vi "SCCAPI Initialize.vi"(8 "error in (no error)":errorcluster, 10 "provider location":string, 11 "providerName":string) -> (0 "error out":errorcluster, 2 "suppCaps":u32)   [LabVIEW 2017, in "NI_SCC.lvlib"]
uses:
  <vilib>/SourceControl/sccapi/NI_SCC.lvlib
  <vilib>/SourceControl/sccapi/SCCAPI SCC Operations.ctl
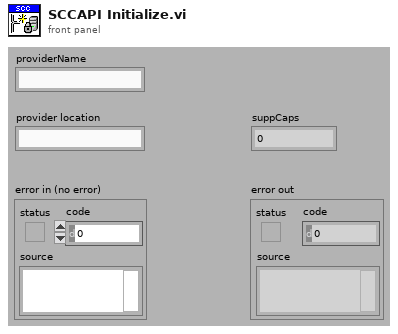
[diagram p1: front panel]
types:
  T1 = typedef "NI_SCC.lvlib/SCCAPI SCC Operations.ctl" = enum16{"Add", "Check In", "Check Out", "Close Project", "Compare Files", "Compare VIs", "Configure Project", "File History", "File Properties", "File Status", "Find All Providers", "Get Advanced Command Options", "Get File Copy", "Get Latest Version", "Get Project Name", "Get StaticVI Path", "Initialize", "Not A Source Control Reference", "Open Project", "Provider Supports Functionality", "Remove", "Run Provider", "Undo Check Out", "Uninitialize", "Is File In Local Path"}
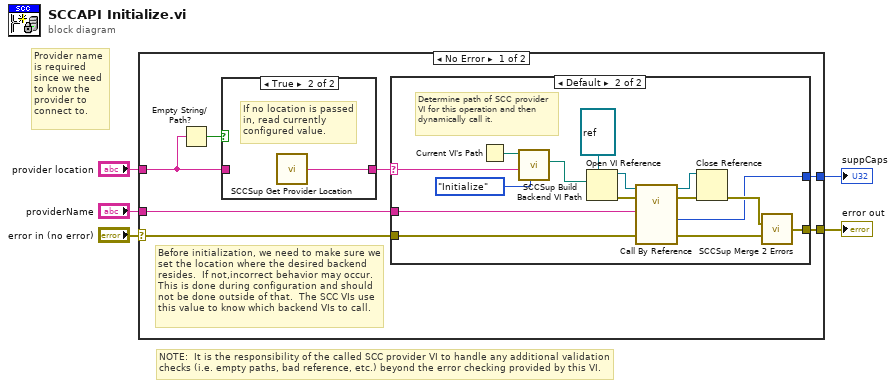
[diagram p0: block diagram]
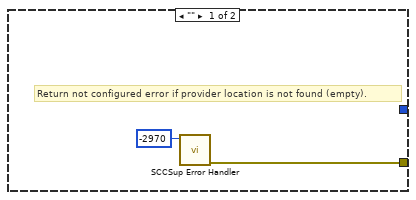
[diagram p3: hidden frame]
diagram:
  # "NOTE:  It is the responsibility of the called SCC provider VI to handle any additional validation checks (i.e. empty paths, bad reference, etc.) beyond the error checking provided by this VI."
  # "Provider name is required since we need to know the provider to connect to."
  n1 = case shown="No Error" "error in (no error)" {
    selector: "error in (no error)" -> [w7 w32]
    tunnel: [w12 w32] -> w4
    tunnel: "providerName" -> [w11 _]
    tunnel: "provider location" -> [w9 _]
    tunnel: [w6 _] -> w1
    frame No Error {
      # "Before initialization, we need to make sure we set the location where the desired backend resides.  If not,incorrect behavior may occur.  This is done during configuration and should not be done outside of that.  The SCC VIs use this value to know which backend VIs to call."
      n2 = Empty String/Path?(string/path=w9) -> (empty?=w10:bool)
      n3 = case shown="True" w10 {
        tunnel: w9 -> [w13 _]
        tunnel: [w13 w14] -> w8
        frame False {
        }
        frame True {
          # "If no location is passed in, read currently configured value."
          n4 = call <vilib>:"SCCSup Get Provider Location.vi"() -> ("provider location"=w14:string)  [unwired: 6 in]
        }
      }
      n5 = case shown="Default" w8 {
        selector: w8 -> [_ w19]
        tunnel: w11 -> [_ w31]
        tunnel: [w15 w30] -> w12
        tunnel: w7 -> [_ w18]
        tunnel: [_ w17] -> w6
        frame "" {
          # "Return not configured error if provider location is not found (empty)."
          n6 = call <vilib>:"SCCSup Error Handler.vi"("scc error code"=-2970 ("code")) -> ("error out"=w15:errorcluster)  [unwired: 10 in]
        }
        frame Default {
          # "Determine path of SCC provider VI for this operation and then dynamically call it."
          n7 = Current VI's Path() -> (path=w22:path)
          n8 = call <vilib>:"SCCSup Build Backend VI Path.vi"("scc operation"=SCCAPI_SCC_Operations."Initialize", "provider location"=w19, "caller path"=w22) -> ("scc backend VI path"=w21:path)  [unwired: 8 in]
          n9 = Open VI Reference(type specifier VI Refnum (for type only)=refnum<vi> refnum, vi path=w21) -> (vi reference=w28:refnum<vi>, error out=w27:errorcluster)  [unwired: 4 in]
          n10 = call-by-ref "?"(reference=w28, error in=w27, "error in (no error)"=w18, "provider name"=w31) -> (reference out=w26:refnum<vi>, error out=w25:errorcluster, 0:"error out"=w23:errorcluster, "suppCaps"=w17:u32)  [unwired: 8 in]
          n11 = Close Reference(reference=w26, error in (no error)=w25) -> (error out=w24:errorcluster)
          n12 = call <vilib>:"SCCSup Merge 2 Errors.vi"("Error IO 1"=w24, "Error IO 2"=w23) -> ("Error IO out"=w30:errorcluster)  [unwired: 13 in]
        }
      }
    }
    frame Error {
    }
  }
  "error out" <- w4
  "suppCaps" <- w1
